vi "Send Chained Command.vi"(8 "error in (no error)":errorcluster, 9 "Imported Commands":string[][](array[string]), 10 "String":string, 11 "VISA Refnum in":refnum<visa-resource-name>) -> (0 "error out":errorcluster, 3 "VISA Refnum out":refnum<visa-resource-name>)   [LabVIEW 2020]
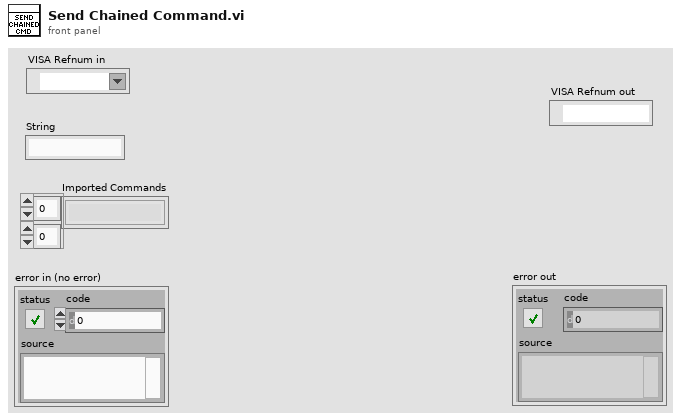
[diagram p1: front panel]
types:
  T1 = typedef "Data Cluster (all strings for now).ctl" = cluster{"Command Name":string, "Command Opcode ":string, "Response Size (bytes)":string}
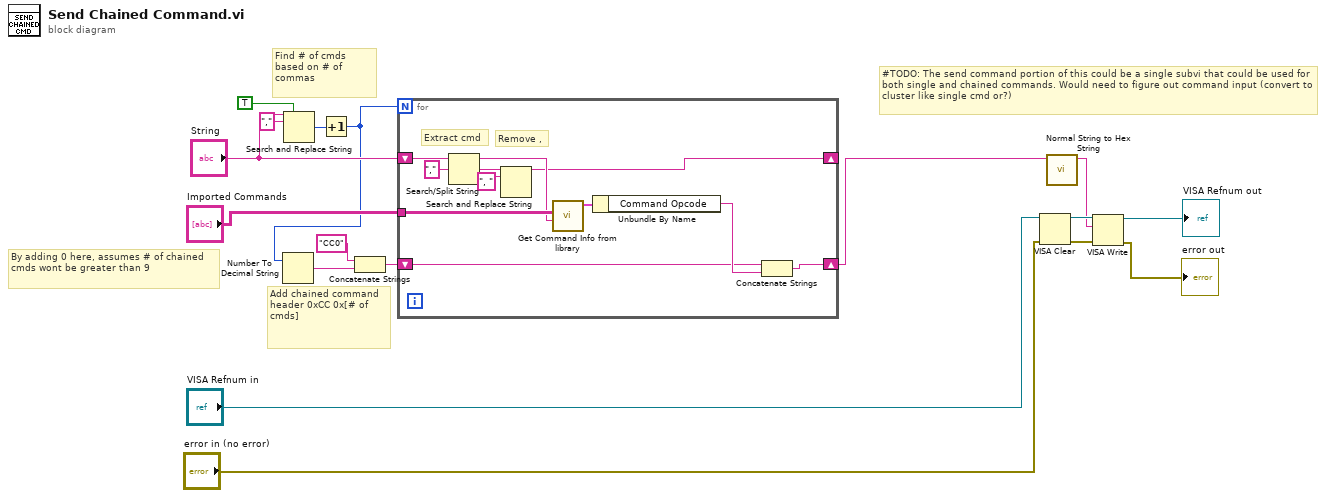
[diagram p0: block diagram]
diagram:
  # "#TODO: The send command portion of this could be a single subvi that could be used for both single and chained commands. Would need to figure out command input (convert to cluster like single cmd or?)"
  # "By adding 0 here, assumes # of chained cmds wont be greater than 9"
  # "Add chained command header 0xCC 0x[# of cmds]"
  # "Find # of cmds based on # of commas"
  n1 = Search and Replace String(replace all?=TRUE ("replace all? (F)"), input string="String", search string=",") -> (number of replacements=w10:i32)  [unwired: 5 in, 3 out]
  n2 = Increment(x=w10) -> (x+1=w9:i32)
  n3 = Number To Decimal String(number=w9) -> (decimal integer string=w14:string)  [unwired: 1 in]
  n4 = Concatenate Strings("CC0", w14) -> (w12:string)
  n5 = for {
    N: w9 -> [_]
    tunnel: "Imported Commands" -> [w24]
    shift-right: [w19] -> w1
    shift-left: w12 -> [w20]
    shift-right: [w18] -> _
    shift-left: "String" -> [w25]
    # "Remove ,"
    # "Extract cmd"
    n6 = Search/Split String(string=w25, search string/char (-)=",") -> (substring before match=w23:string, match + rest of string=w28:string)  [unwired: 1 in, 1 out]
    n7 = Search and Replace String(input string=w28, search string=", ") -> (result string=w18:string)  [unwired: 6 in, 3 out]
    n8 = call "Get Command Info from library.vi"("Step"=w23, "Imported Commands"=w24) -> ("Data cluster"=w22:T1)  [unwired: 9 in]
    n9 = Unbundle By Name(w22) -> ("Command Opcode"=w21:string)
    n10 = Concatenate Strings(w20, w21) -> (w19:string)
  }
  n11 = VISA Clear(VISA resource name="VISA Refnum in", error in (no error)="error in (no error)") -> (VISA resource name out=w5:refnum<visa-resource-name>, error out=w6:errorcluster)
  n12 = call "Normal String to Hex String.vi"("Command Opcode"=w1) -> ("Hex String"=w4:string)  [unwired: 10 in]
  n13 = VISA Write(VISA resource name=w5, write buffer=w4, error in (no error)=w6) -> (VISA resource name out=→"VISA Refnum out":refnum<visa-resource-name>, error out=→"error out":errorcluster)  [unwired: 1 out]
